vi "Tektronix DPO MSO 2000 4000 Series Acquire Digital Waveform Example.vi"() -> ()   [LabVIEW 2017]
doc: "This example illustrates how to use autosetup and acquire a waveform on a single digital channel using the following steps:\n\n1. Specify a valid VISA session. \n2. Specify a digital channel. \n3. Specify a time-out value for reading waveform.\n4. Run the VI. The graph displays the waveform you acquire. \n\n<B>Note:</B>\n- This VI does not work with DPO series oscilloscopes.\n- LabVIEW versions higher than 7.1 might display the data differently."
uses:
  <instrlib>/Tektronix DPO MSO 2000 4000 Series/Public/Data/Read (Single Digital Waveform).vi
  <instrlib>/Tektronix DPO MSO 2000 4000 Series/Tektronix DPO MSO 2000 4000 Series.lvlib
panel:
  in  "Digital Channel (14: Channel 1)":u16(ring)=14 items=["Digital Channel 0"=14, "Digital Channel 1"=15, "Digital Channel 2"=16, "Digital Channel 3"=17, "Digital Channel 4"=18, "Digital Channel 5"=19, "Digital Channel 6"=20, "Digital Channel 7"=21, "Digital Channel 8"=22, "Digital Channel 9"=23, "Digital Channel 10"=24, "Digital Channel 11"=25, "Digital Channel 12"=26, "Digital Channel 13"=27, "Digital Channel 14"=28, "Digital Channel 15"=29]
  out "Digital Waveform":digitalwaveform(graph)
  in  "Maximum Time (10000ms)":u32=10000
  in  "VISA Resource Name":refnum<visa-resource-name>
  # "(C) 2006 - 2016. National Instruments Corporation. ALL RIGHTS RESERVED."
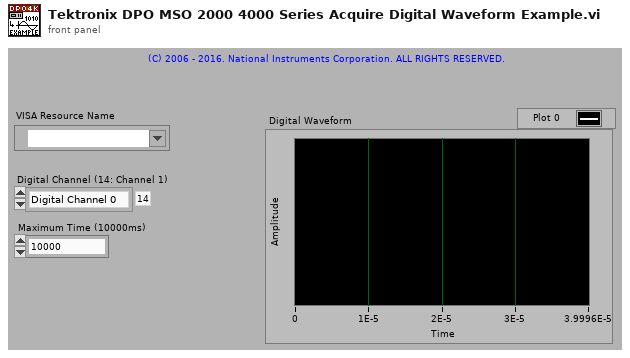
[diagram p1: front panel]
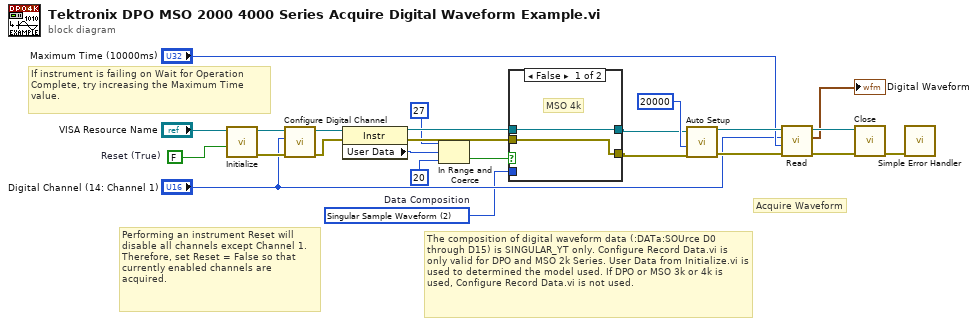
[diagram p0: block diagram]
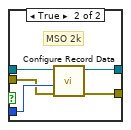
[diagram p2: hidden frame]
diagram:
  w11 = u16 2 items=["Composite Sample Waveform", "Composite Peak Detect Waveform", "Singular Sample Waveform"]  # Data Composition
  w20 = FALSE  # Reset (True)
  # "The composition of digital waveform data (:DATa:SOUrce D0 through D15) is SINGULAR_YT only. Configure Record Data.vi is only valid for DPO and MSO 2k Series. User Data from Initialize.vi is used to determined the model used. If DPO or MSO 3k or 4k is used, Configure Record Data.vi is not used."
  # "If instrument is failing on Wait for Operation Complete, try increasing the Maximum Time value."
  # "Performing an instrument Reset will disable all channels except Channel 1. Therefore, set Reset = False so that currently enabled channels are acquired."
  # "Acquire Waveform"
  n1 = call <instrlib>:"Initialize.vi"("Reset (True)"=w20, "VISA resource name"="VISA Resource Name") -> ("error out"=w13:errorcluster, "VISA resource name out"=w14:refnum<visa-resource-name>)  [unwired: 8 in]
  n2 = call <instrlib>:"Configure Digital Channel.vi"("error in (no error)"=w13, "Digital Channel (14: Digital Channel 0)"="Digital Channel (14: Channel 1)", "VISA resource name"=w14) -> ("error out"=w7:errorcluster, "VISA resource name out"=w8:refnum<visa-resource-name>)  [unwired: 7 in]
  n3 = property class="Instr"(reference=w8, error in=w7) -> (reference out=w10:refnum<visa-resource-name>, error out=w9:errorcluster, "User Data"=w4:u32)
  n4 = In Range and Coerce(upper limit=u32 27, x=w4, lower limit=u32 20) -> (In Range?=w1:bool)  [unwired: 1 out]
  n5 = case shown="False" w1 {
    tunnel: [w26 w31] -> w6
    tunnel: [w25 w30] -> w5
    tunnel: w11 -> [_ w29]
    tunnel: w10 -> [w26 w28]
    tunnel: w9 -> [w25 w27]
    frame False {
      # "MSO 4k"
    }
    frame True {
      # "MSO 2k"
      n6 = call <instrlib>:"Configure Record Data.vi"("error in (no error)"=w27, "Data Composition (0: Composite Sample Waveform)"=w29, "VISA resource name"=w28) -> ("error out"=w30:errorcluster, "VISA resource name out"=w31:refnum<visa-resource-name>)  [unwired: 7 in]
    }
  }
  n7 = call <instrlib>:"Auto Setup.vi"("error in (no error)"=w5, "Maximum Time (10000ms)"=u32 20000, "VISA resource name"=w6) -> ("error out"=w17:errorcluster, "VISA resource name out"=w19:refnum<visa-resource-name>)  [unwired: 7 in]
  n8 = call-poly <instrlib>:"Read.vi"("error in (no error)"=w17, "Maximum Time (10000ms)"="Maximum Time (10000ms)", "Digital Channel (14: Digital Channel D0)"="Digital Channel (14: Channel 1)", "VISA resource name"=w19) -> ("error out"=w21:errorcluster, "Digital Waveform"=→"Digital Waveform":digitalwaveform, "VISA resource name out"=w22:refnum<visa-resource-name>)  [unwired: 5 in]
  n9 = call <instrlib>:"Close.vi"("error in (no error)"=w21, "VISA resource name"=w22) -> ("error out"=w23:errorcluster)  [unwired: 9 in]
  n10 = call <vilib>:"Simple Error Handler.vi"("error in (no error)"=w23) -> ()  [unwired: 4 in, 5 out]
